vi "Gantry Camera to Physical Coordinates.vi"(8 "error in":errorcluster, 10 "Image Coordinate":refnum<class "Vec3d Class.lvclass">, 11 "Physical Image":T1) -> (0 "error out":errorcluster, 2 "Global Coordinate":refnum<class "Vec3d Class.lvclass">, 3 "Physical Image out":T1)   [LabVIEW 2011]
doc: "Given a Physical Image, and a set of x,y coordinates of a point within that image, find the physical location of that point; meaning the coordinates that put the gantry camera directly over the point and in focus.\n\nx ranges from (0->1)\ny ranges from (0->1)\n(x,y)=(0,0) is the top-left corner of the image"
uses:
  Vec3d Class/Vec3d Class.lvclass
  Type Definitions/Physical Image.ctl
  <vilib>/vision/Image Controls.llb/IMAQ Image.ctl
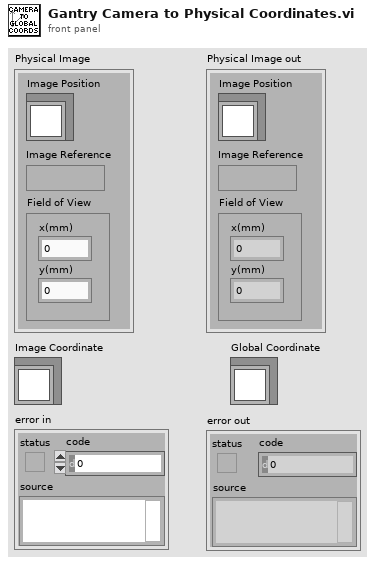
[diagram p1: front panel]
types:
  T1 = typedef "Physical Image.ctl" = cluster{"Image Position":refnum<class "Vec3d Class.lvclass">, "Image Reference":T2, "Field of View":cluster{"x(mm)":dbl, "y(mm)":dbl}}
  T2 = typedef "IMAQ Image.ctl" = refnum<image>
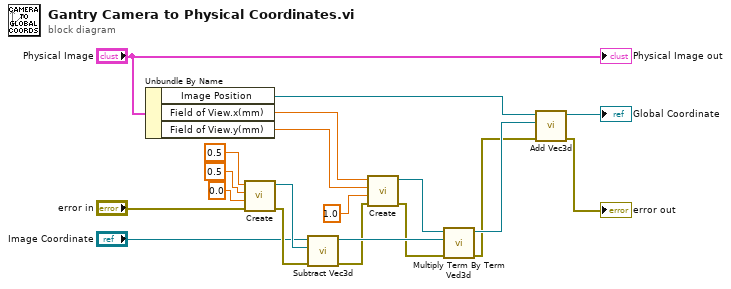
[diagram p0: block diagram]
diagram:
  n1 = Unbundle By Name("Physical Image") -> ("Image Position"=w6:refnum<class "Vec3d Class.lvclass">, "Field of View.x(mm)"=w5:dbl, "Field of View.y(mm)"=w4:dbl)
  n2 = call "Create.vi"("error in"="error in", "Z"=0.0, "Y"=0.5, "X"=0.5) -> ("error out"=w12:errorcluster, "Vec3d Class out"=w2:refnum<class "Vec3d Class.lvclass">)  [unwired: 6 in]
  n3 = call "Subtract Vec3d.vi"("error in (no error)"=w12, "Vec3d in 2"=w2, "Vec3d in 1"="Image Coordinate") -> ("error out"=w11:errorcluster, "Vec3d Class out"=w16:refnum<class "Vec3d Class.lvclass">)  [unwired: 7 in]
  n4 = call "Create.vi"("error in"=w11, "Z"=1.0, "Y"=w4, "X"=w5) -> ("error out"=w10:errorcluster, "Vec3d Class out"=w20:refnum<class "Vec3d Class.lvclass">)  [unwired: 6 in]
  n5 = call-dynamic "Multiply Term By Term Ved3d.vi"("error in"=w10, "Vec3d in 2"=w16, "Vec3d in 1"=w20) -> ("error out"=w9:errorcluster, "Vec3d Class out"=w18:refnum<class "Vec3d Class.lvclass">)  [unwired: 7 in]
  n6 = call-dynamic "Add Vec3d.vi"("error in (no error)"=w9, 10:"Vec3d Class in"=w18, 11:"Vec3d Class in"=w6) -> ("error out"=→"error out":errorcluster, "Vec3d Class out"=→"Global Coordinate":refnum<class "Vec3d Class.lvclass">)  [unwired: 7 in]
  "Physical Image out" <- "Physical Image"
